vi "Modify Name.vi"(8 "error in (no error)":errorcluster, 10 "Name Edit Config":T1, 11 "Path in":path) -> (0 "error out":errorcluster, 2 "Formatted name":string, 3 "Dup Path out":path)   [LabVIEW 2019, in "AutoMenuCreator.lvlib"]
uses:
  AutoMenuCreator.lvlib
  Ctl/Ctl_Config_Name Edit.ctl
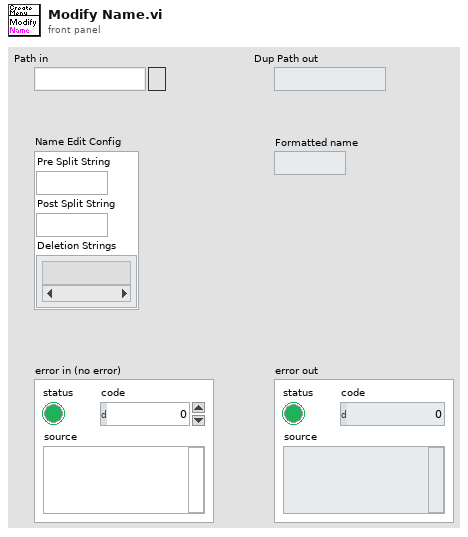
[diagram p1: front panel]
types:
  T1 = typedef "AutoMenuCreator.lvlib/Ctl_Config_Name Edit.ctl" = cluster{"Pre Split String":string, "Post Split String":string, "Deletion Strings":string[]}
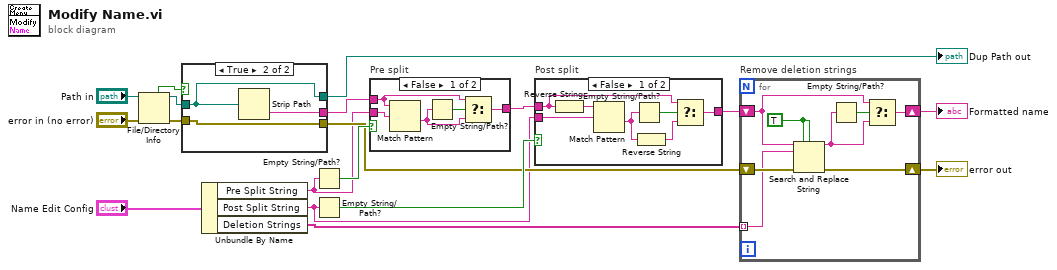
[diagram p0: block diagram]
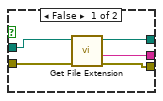
[diagram p2: hidden frame]
diagram:
  n1 = File/Directory Info(path="Path in", error in="error in (no error)") -> (path out=w4:path, directory=w1:bool, error out=w2:errorcluster)  [unwired: 4 out]
  n2 = case shown="True" w1 {
    tunnel: [w23 w24] -> w18
    tunnel: [w22 w26] -> w17
    tunnel: [w21 w25] -> w11
    tunnel: w4 -> [w20 w26]
    tunnel: w2 -> [w19 w25]
    frame False {
      n3 = call <vilib>:"Get File Extension.vi"("error in (no error)"=w19, "file"=w20) -> ("error out"=w21:errorcluster, "filename without extension"=w23:string, "dup file"=w22:path)  [unwired: 5 in, 2 out]
    }
    frame True {
      n4 = Strip Path(path=w26) -> (name=w24:string)  [unwired: 1 out]
    }
  }
  "Dup Path out" <- w17
  n5 = Unbundle By Name("Name Edit Config") -> ("Pre Split String"=w7:string, "Post Split String"=w6:string, "Deletion Strings"=w8:string[])
  n6 = Empty String/Path?(string/path=w7) -> (empty?=w16:bool)
  n7 = Empty String/Path?(string/path=w6) -> (empty?=w15:bool)
  n8 = case "Pre split" shown="False" w16 {
    tunnel: [w31 w32] -> w14
    tunnel: w18 -> [w29 w32]
    tunnel: w7 -> [w27 _]
    frame False {
      n9 = Match Pattern(string=w29, regular expression=w27) -> (after substring=w30:string)  [unwired: 1 in, 3 out]
      n10 = Empty String/Path?(string/path=w30) -> (empty?=w28:bool)
      n11 = Select(t=w29, s=w28, f=w30) -> (s? t:f=w31:string)
    }
    frame True {
    }
  }
  n12 = case "Post split" shown="False" w15 {
    tunnel: [w33 w40] -> w13
    tunnel: w14 -> [w35 w40]
    tunnel: w6 -> [w37 _]
    frame False {
      n13 = Reverse String(1:w35) -> (0:w36:string)
      n14 = Match Pattern(string=w36, regular expression=w37) -> (after substring=w39:string)  [unwired: 1 in, 3 out]
      n15 = Empty String/Path?(string/path=w39) -> (empty?=w38:bool)
      n16 = Reverse String(1:w39) -> (0:w34:string)
      n17 = Select(t=w35, s=w38, f=w34) -> (s? t:f=w33:string)
    }
    frame True {
    }
  }
  n18 = for "Remove deletion strings" {
    shift-right: [w41] -> w12
    shift-left: w13 -> [w43]
    shift-right: [w48] -> w10
    shift-left: w11 -> [w47]
    tunnel: w8 -> [w46] mode=indexing
    w45 = TRUE ("ignore case? (F)")
    n19 = Search and Replace String(replace all?=w45, case sensitive?=w45, input string=w43, search string=w46, error in=w47) -> (result string=w42:string, error out=w48:errorcluster)  [unwired: 3 in, 2 out]
    n20 = Empty String/Path?(string/path=w42) -> (empty?=w44:bool)
    n21 = Select(t=w43, s=w44, f=w42) -> (s? t:f=w41:string)
  }
  "error out" <- w10
  "Formatted name" <- w12
